vi "Remove Empty Path.vi"(5 "instr vi paths in":path[](array[path])) -> (2 "instr vi paths out":path[](array[path]))   [LabVIEW 2021, in "Path Functions.lvlib"]
uses:
  Path Functions.lvlib
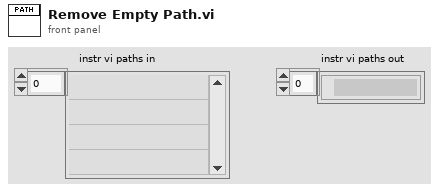
[diagram p1: front panel]
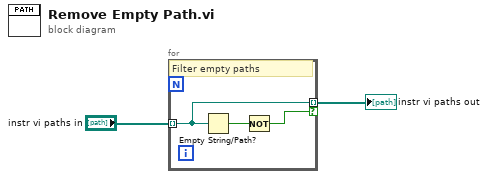
[diagram p0: block diagram]
diagram:
  n1 = for {
    tunnel: "instr vi paths in" -> [w4] mode=indexing
    tunnel: [w4] -> w2 mode=indexing if=w3
    # "Filter empty paths"
    n2 = Empty String/Path?(string/path=w4) -> (empty?=w5:bool)
    n3 = Not(x=w5) -> (.not. x?=w3:bool)
  }
  "instr vi paths out" <- w2
